vi "Text.vi"(1 "Input 2":string, 2 "Input 1":string) -> (0 "Result":string)   [LabVIEW 2019]
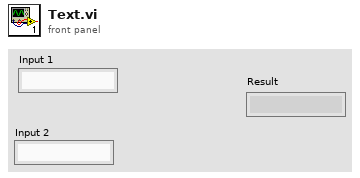
[diagram p1: front panel]
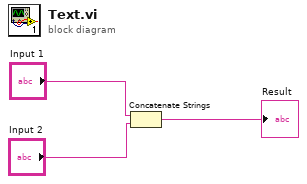
[diagram p0: block diagram]
diagram:
  n1 = Concatenate Strings("Input 1", "Input 2") -> (→"Result":string)
